vi "waitBLResponse.vi"(5 "timout(ms)":u32=5000, 7 "Response":T1=520224768 items=["LM_API_UPD_PING"=520224768, "LM_API_UPD_DOWNLOAD"=520224832, "LM_API_UPD_SEND_DATA"=520224896, "LM_API_UPD_RESET"=520224960, "LM_API_UPD_ACK"=520225024, "LM_API_UPD_REQUEST"=520225152], 8 "Error in":errorcluster {"code" format="%.0x"}, 11 "ObjHandle in":T3) -> (0 "Error out":errorcluster {"code" format="%.0x"}, 1 "msgData":T2[](array[typedef]) {"Data" format="%.0x"; "ArbitrationId" format="%.0x"; "Timestamp" format="%<%I:%M:%S%3u %p\n%m/%d/%Y>T"}, 2 "msgCount":u32, 3 "ObjHandle out":T3)   [LabVIEW 2017]
uses:
  <vilib>/nican/nican.llb/xobjhandle.ctl
  <vilib>/nican/nican.llb/CanFrameTimed.ctl
  LM_API_UPD.ctl
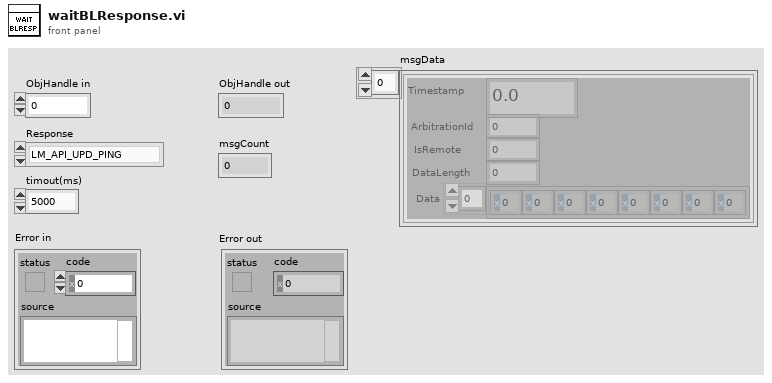
[diagram p1: front panel]
types:
  T1 = typedef "LM_API_UPD.ctl" = u32
  T2 = typedef "CanFrameTimed.ctl" = cluster{"Timestamp":dbl, "ArbitrationId":u32, "IsRemote":u8, "DataLength":u8, "Data":u8[]}
  T3 = typedef "xobjhandle.ctl" = u32
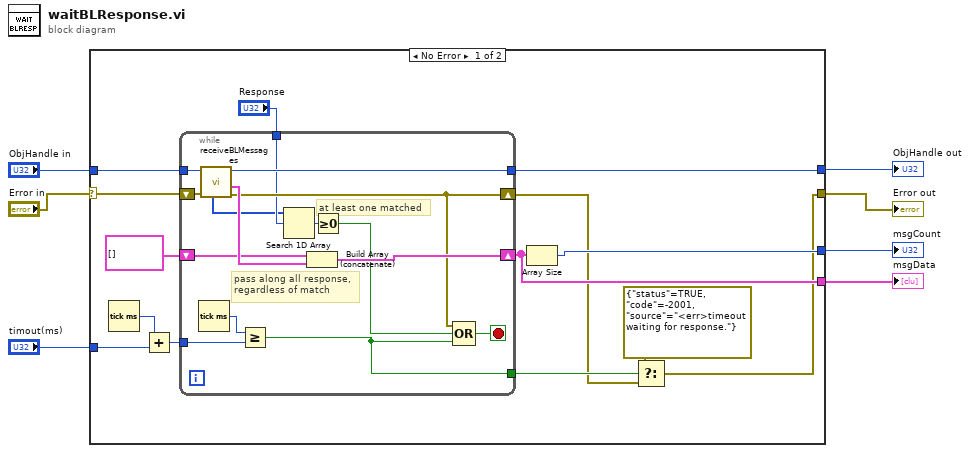
[diagram p0: block diagram]
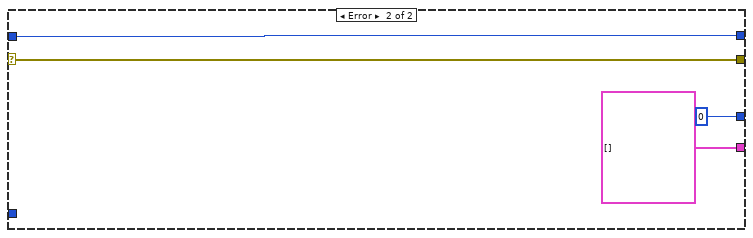
[diagram p2: hidden frame]
diagram:
  n1 = case shown="No Error" "Error in" {
    selector: "Error in" -> [w20 w39]
    tunnel: "ObjHandle in" -> [w21 w40]
    tunnel: [w13 w40] -> w6
    tunnel: [w8 w39] -> w4
    tunnel: [w14 T2[] [] ("Data")] -> w3
    tunnel: [w15 u32 0 ("ActualDataSize (Frames)")] -> w2
    tunnel: "timout(ms)" -> [w18 _]
    frame No Error {
      n2 = Tick Count (ms)() -> (millisecond timer value=w19:u32)
      n3 = Add(x=w19, y=w18) -> (x+y=w17:u32)
      n4 = while {
        tunnel: w21 -> [w36]
        tunnel: w17 -> [w33]
        shift-right: [w30] -> w14
        shift-left: T2[] [] ("msgData") -> [w31]
        tunnel: [w29] -> w13
        tunnel: "Response" -> [w24]
        tunnel: [w26] -> w11
        shift-right: [w25] -> w10
        shift-left: w20 -> [w35]
        stop <- w27 stop-if-true
        # "pass along all response,\nregardless of match"
        # "at least one matched"
        n5 = Tick Count (ms)() -> (millisecond timer value=w34:u32)
        n6 = call "receiveBLMessages.vi"("Error in"=w35, "ObjHandle in"=w36) -> ("Error out"=w25:errorcluster, "msgData"=w32:T2[], "ObjHandle out"=w29:T3, "msgIDs"=w23:u32[])  [unwired: 5 in, 1 out]
        n7 = Greater Or Equal?(x=w34, y=w33) -> (x >= y?=w26:bool)
        n8 = Search 1D Array(1D array=w23, element=w24) -> (index of element=w28:i32)  [unwired: 1 in]
        n9 = Build Array (concatenate)(w31, w32) -> (w30:T2[])
        n10 = Greater Or Equal To 0?(x=w28) -> (x >= 0?=w22:bool)
        n11 = Compound Arithmetic op=OR(w25, w22, w26) -> (w27:bool)
      }
      n12 = Array Size(array=w14) -> (size(s)=w15:i32)
      n13 = Select(t=errorcluster {"status"=TRUE, "code"=-2001, "source"="<err>timeout waiting for response."}, s=w11, f=w10) -> (s? t:f=w8:errorcluster)
    }
    frame Error {
    }
  }
  "ObjHandle out" <- w6
  "Error out" <- w4
  "msgData" <- w3
  "msgCount" <- w2
